vi "Esercitazione 8 - Acquisizione ed elaborazione audio (easy).vi"() -> ()   [LabVIEW 2018]
uses:
  <vilib>/measure/maspectr.llb/FFT Spectrum (Mag-Phase) for N Chan.vi
  <vilib>/Waveform/WDTOps.llb/WDT Index Channel DBL.vi
  <vilib>/measure/NI_MAPro.lvlib
panel:
  out "Waveform Graph 2":cluster{"f0":dbl, "df":dbl, "magnitude":dbl[]}[](graph)
  out "Waveform Graph":cluster{"f0":dbl, "df":dbl, "magnitude":dbl[]}[](graph)
  out "dt":dbl
  out "t0":timestamp
  out "Data":dynamicdata(graph)
  in  "Duration (s)":dbl=5.0
  # "data acquisizione primo campione"
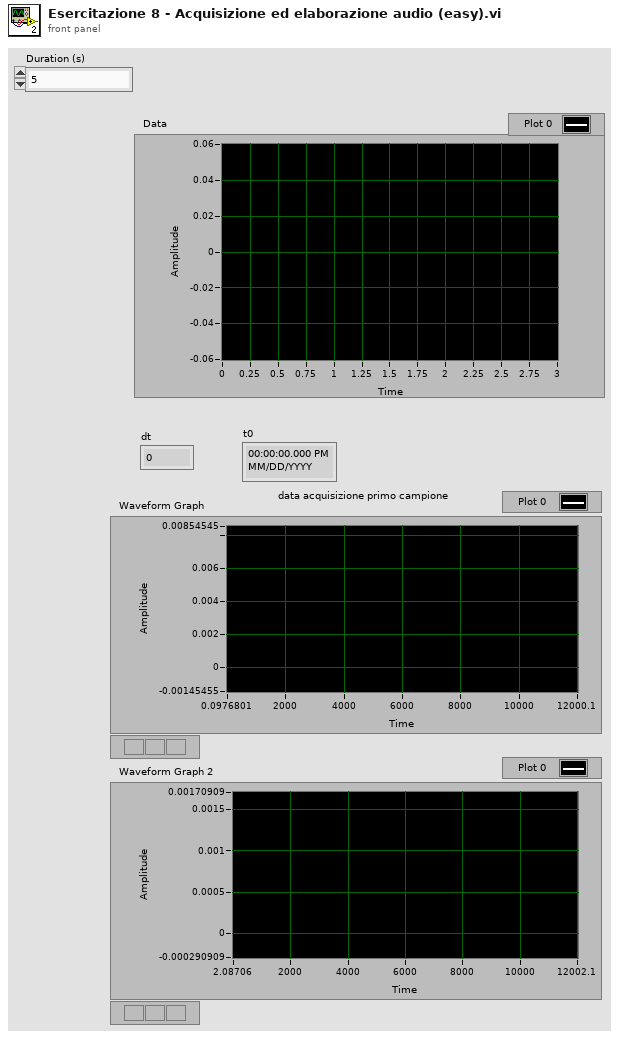
[diagram p1: front panel]
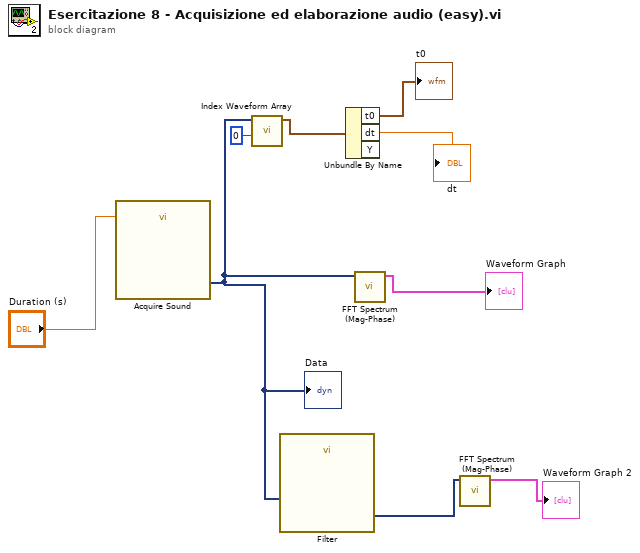
[diagram p0: block diagram]
diagram:
  n1 = call "Acquire Sound"("Duration (s)"="Duration (s)") -> ("Data"=w3:dynamicdata)  [unwired: 17 in, 1 out]
  "Data" <- w3
  n2 = call-poly <vilib>:"Index Waveform Array.vi"("index"=0, "waveform array"=w3) -> ("waveform"=w7:waveform(dbl))  [unwired: 8 in, 1 out]
  n3 = call "Filter"("Signal"=w3) -> ("Filtered Signal"=w2:dynamicdata)  [unwired: 9 in, 1 out]
  n4 = Unbundle By Name(w7) -> ("t0"=→"t0":timestamp, "dt"=→"dt":dbl)  [unwired: 1 out]
  n5 = call-poly <vilib>:"FFT Spectrum (Mag-Phase).vi"("time signals"=w3) -> ("magnitudes"=→"Waveform Graph":cluster{"f0":dbl, "df":dbl, "magnitude":dbl[]}[])  [unwired: 6 in, 4 out]
  n6 = call-poly <vilib>:"FFT Spectrum (Mag-Phase).vi"("time signals"=w2) -> ("magnitudes"=→"Waveform Graph 2":cluster{"f0":dbl, "df":dbl, "magnitude":dbl[]}[])  [unwired: 6 in, 4 out]
